vi "RT_Read_Websocket.vi"(10 "SettingsActuators":refnum<notifier>, 11 "WebSocket Server in":refnum<class "WebSocket Server.lvclass">) -> (0 "process error":errorcluster, 1 "socket error":errorcluster, 3 "WebSocket Server out":refnum<class "WebSocket Server.lvclass">)   [LabVIEW 2019]
uses:
  Settings_Actuators.ctl
  <vilib>/MediaMongrels Ltd/WebSockets/WebSockets/WebSocket Server/WebSocket Server.lvclass
  <vilib>/addons/_JKI.lib/Serialization/JSON/JKI JSON Serialization.lvlib
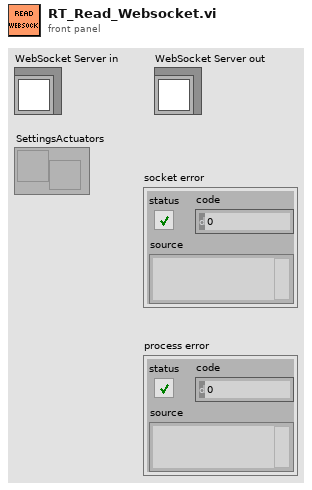
[diagram p1: front panel]
types:
  T1 = typedef "Settings_Actuators.ctl" = cluster{"Kiuas_Button_LED":bool, "Loyly_Button_LED":bool, "Loyly_Valve_Enable":bool, "Loyly_Valve":bool, "Aromi_Button_LED":bool, "Aromi_Pump_Enable":bool, "Aromi_Pump":bool, "Aromi_Pump_Direction":bool, "Aromi_Pump_Cycle":u32}
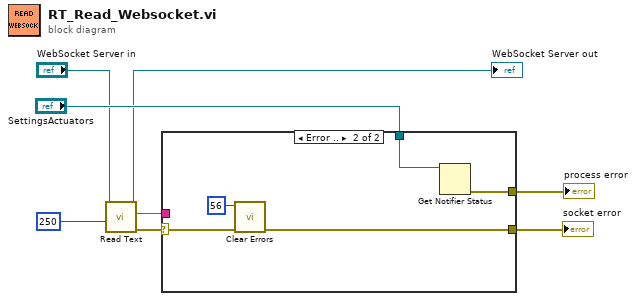
[diagram p0: block diagram]
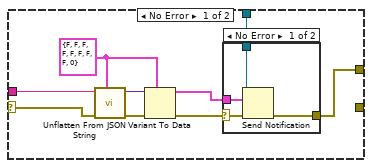
[diagram p2: hidden frame]
diagram:
  n1 = call-dynamic "Read Text.vi"("timeout ms (5000)"=250, "WebSocket in"="WebSocket Server in") -> ("error out"=w3:errorcluster, "Data"=w7:string, "WebSocket out"=→"WebSocket Server out":refnum<class "WebSocket Server.lvclass">)  [unwired: 7 in]
  n2 = case shown="Error .." w3 {
    selector: w3 -> [w10 w26]
    tunnel: "SettingsActuators" -> [w12 w24]
    tunnel: w7 -> [w11 _]
    tunnel: [_ w25] -> w2
    tunnel: [w9 w23] -> w1
    frame No Error {
      w14 = T1 {"Kiuas_Button_LED"=FALSE, "Loyly_Button_LED"=FALSE, "Loyly_Valve_Enable"=FALSE, "Loyly_Valve"=FALSE, "Aromi_Button_LED"=FALSE, "Aromi_Pump_Enable"=FALSE, "Aromi_Pump"=FALSE, "Aromi_Pump_Direction"=FALSE, "Aromi_Pump_Cycle"=0} ("notification")
      n3 = call <vilib>:"Unflatten From JSON String.vi"("Type and Defaults"=w14, "error in (no error)"=w10, "JSON String"=w11) -> ("error out"=w15:errorcluster, "Variant"=w13:variant)  [unwired: 7 in]
      n4 = Variant To Data(error in=w15, type=w14, Variant=w13) -> (data=w16:T1, error out=w17:errorcluster)
      n5 = case shown="No Error" w17 {
        selector: w17 -> [w19 w22]
        tunnel: w12 -> [w21 _]
        tunnel: w16 -> [w20 _]
        tunnel: [w18 w22] -> w9
        frame No Error {
          n6 = Send Notification(notification=w20, notifier=w21, error in (no error)=w19) -> (error out=w18:errorcluster)  [unwired: 1 out]
        }
        frame Error {
        }
      }
    }
    frame Error {
      n7 = call <vilib>:"Clear Errors.vi"("error in (no error)"=w26, "specific error code to clear (0: all)"=56) -> ("error out"=w25:errorcluster)  [unwired: 4 in, 1 out]
      n8 = Get Notifier Status(notifier=w24) -> (error out=w23:errorcluster)  [unwired: 1 in, 4 out]
    }
  }
  "process error" <- w1
  "socket error" <- w2
